vi "PostCopyScripting.vi"(10 "MetaDataObj":refnum<class "MetaDataObj.lvclass">, 11 "User Project":refnum<vi>) -> ()   [LabVIEW 2013, in "FixedChannelTBModuleDecideFeatures.lvclass"]
uses:
  FixedChannelTBModuleDecideFeatures.lvclass
  <resource>/dialog/NewProjectWizard/MetaDataObj/MetaDataObj.lvclass
  FixedChannelTBModuleDecideFeatures.lvclass/FixedChannelTBModuleDecideFeatures.ctl
  Read component name.vi
  Read Channel Specification.vi
  <resource>/dialog/NewProjectWizard/MetaDataObj/Accessors/Read Project Path.vi
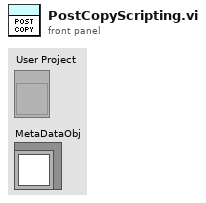
[diagram p1: front panel]
types:
  T1 = typedef "channel configuration.ctl" = cluster{"Name":string, "channel classification":T2, "data type":T3}
  T2 = typedef "TBM channel.lvclass/channel classification.ctl" = enum16{"input data", "output data", "processing parameter", "processing result"}
  T3 = typedef "tag bus.lvlib/tag descriptor.lvclass/Data Type.ctl" = enum16{"Double", "Single", "I64", "I32", "I16", "I8", "U64", "U32", "U16", "U8", "Boolean", "String", "Array of Double", "Array of Single", "Array of I64", "Array of I32", "Array of I16", "Array of I8", "Array of U64", "Array of U32", "Array of U16", "Array of U8", "Array of Boolean", "Array of String"}
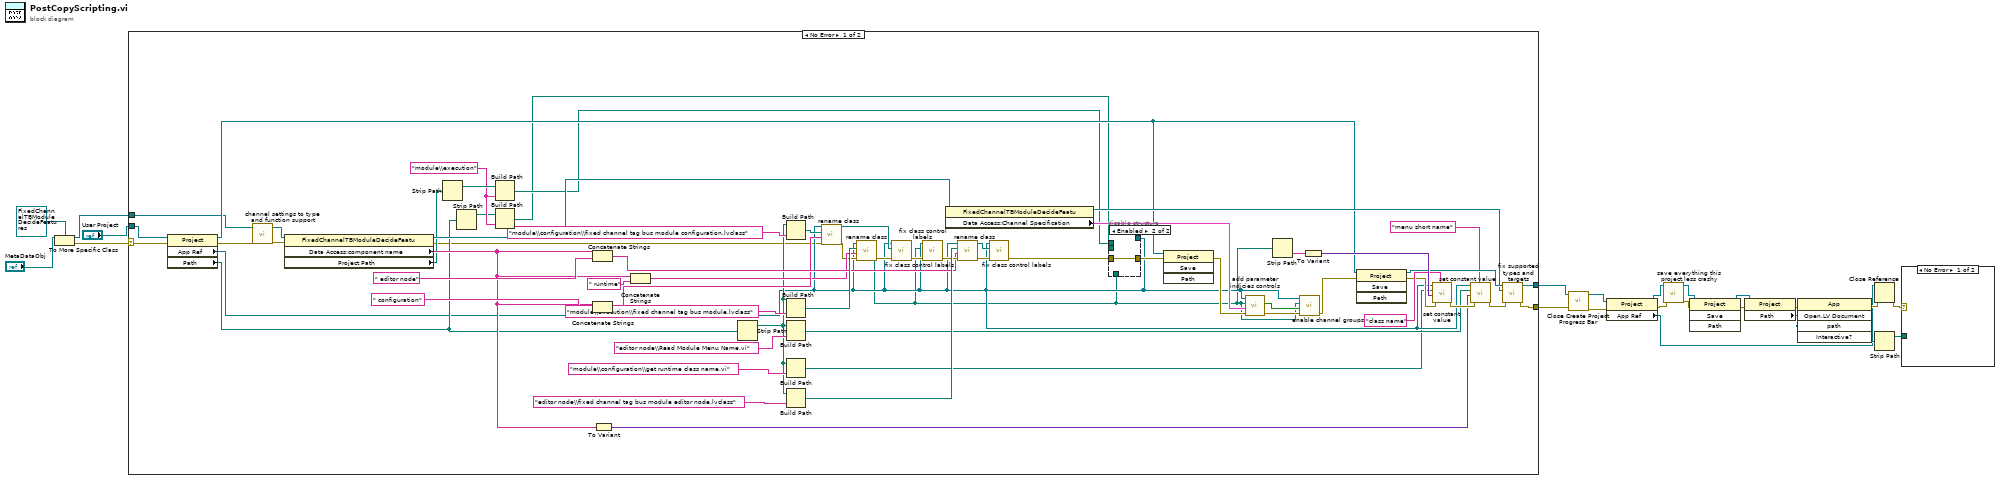
[diagram p0: block diagram]
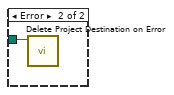
[diagram p2: hidden frame]
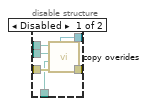
[diagram p3: hidden frame]
diagram:
  n1 = To More Specific Class(target class=refnum<class "FixedChannelTBModuleDecideFeatures.lvclass"> refnum ("DecideProjectFeatures.lvclass"), reference="MetaDataObj") -> (specific class reference=w12:refnum<class "FixedChannelTBModuleDecideFeatures.lvclass">, error out=w19:errorcluster)  [unwired: 1 in]
  n2 = case shown="No Error" w19 {
    selector: w19 -> [w24 w91]
    tunnel: [w63 w92] -> w1
    tunnel: "User Project" -> [w23 w92]
    tunnel: [w64 w91] -> w4
    tunnel: w12 -> [w26 _]
    frame No Error {
      w39 = "module\\execution"
      n3 = property class="Project"(reference=w23, error in=w24) -> (reference out=w42:refnum<vi>, error out=w25:errorcluster, "App Ref"=w31:refnum<vi>, "Path"=w37:path)
      n4 = call "channel settings to type and function support.vi"("error in"=w25, "FixedChannelTBModuleDecideFeatures in"=w26) -> ("error out"=w28:errorcluster, "FixedChannelTBModuleDecideFeatures out"=w27:refnum<class "FixedChannelTBModuleDecideFeatures.lvclass">)  [unwired: 8 in]
      n5 = property class="FixedChannelTBModuleDecideFeatu"(reference=w27, error in=w28) -> (reference out=w79:refnum<class "FixedChannelTBModuleDecideFeatures.lvclass">, error out=w29:errorcluster, "Data Access:component name"=w51:string, "Project Path"=w41:path)
      n6 = Strip Path(path=w41) -> (stripped path=w40:path)  [unwired: 1 out]
      n7 = Strip Path(path=w37) -> (stripped path=w36:path)  [unwired: 1 out]
      n8 = Build Path(base path=w40, name or relative path=w39) -> (appended path=w38:path)
      n9 = Build Path(base path=w36, name or relative path=w39) -> (appended path=w34:path)
      n10 = Concatenate Strings(w51, " editor node" ("string")) -> (w65:string)
      n11 = Concatenate Strings(w51, " configuration" ("string")) -> (w61:string)
      n12 = To Variant(anything=w51) -> (Variant=w57:variant)
      n13 = Concatenate Strings(w51, " runtime" ("string")) -> (w53:string)
      n14 = Strip Path(path=w37) -> (stripped path=w52:path)  [unwired: 1 out]
      n15 = Build Path(base path=w52, name or relative path="module\\configuration\\fixed channel tag bus module configuration.lvclass") -> (appended path=w49:path)
      n16 = Build Path(base path=w52, name or relative path="module\\execution\\fixed channel tag bus module.lvclass") -> (appended path=w81:path)
      n17 = Build Path(base path=w52, name or relative path="editor node\\Read Module Menu Name.vi") -> (appended path=w55:path)
      n18 = Build Path(base path=w52, name or relative path="module\\configuration\\get runtime class name.vi") -> (appended path=w22:path)
      n19 = Build Path(base path=w52, name or relative path="editor node\\fixed channel tag bus module editor node.lvclass") -> (appended path=w70:path)
      n20 = call "rename class.vi"("error in"=w29, "new name"=w61, "class path"=w49, "Application in"=w31) -> ("error out"=w50:errorcluster, "New Library Path"=w48:path)  [unwired: 6 in]
      n21 = call "rename class.vi"("error in"=w50, "new name"=w53, "class path"=w81, "Application in"=w31) -> ("error out"=w73:errorcluster, "New Library Path"=w30:path)  [unwired: 6 in]
      n22 = call "fix class control labels.vi"("error in"=w73, "class to load"=w48, "Application in"=w31) -> ("error out"=w72:errorcluster)  [unwired: 8 in]
      n23 = call "fix class control labels.vi"("error in"=w72, "class to load"=w30, "Application in"=w31) -> ("error out"=w67:errorcluster)  [unwired: 8 in]
      n24 = property class="FixedChannelTBModuleDecideFeatu"(reference=w79) -> (reference out=w47:refnum<class "FixedChannelTBModuleDecideFeatures.lvclass">, "Data Access:Channel Specification"=w46:T1[])  [unwired: 1 in, 1 out]
      n25 = call "rename class.vi"("error in"=w67, "new name"=w65, "class path"=w70, "Application in"=w31) -> ("error out"=w68:errorcluster, "New Library Path"=w69:path)  [unwired: 6 in]
      n26 = call "fix class control labels.vi"("error in"=w68, "class to load"=w69, "Application in"=w31) -> ("error out"=w32:errorcluster)  [unwired: 8 in]
      n27 = disable-structure shown="Enabled" {
        disable-tunnel: w38 -> [w89 _]
        disable-tunnel: w34 -> [w88 _]
        disable-tunnel: [w87 w90] -> w33
        disable-tunnel: w32 -> [w86 w90]
        disable-tunnel: w31 -> [w85 _]
        disable-tunnel: w30 -> [w84 _]
        frame Disabled {
          n28 = call "copy overides.vi"("application reference (local)"=w85, "error in"=w86, "New class path"=w84, "New path"=w88, "Old Path"=w89) -> ("error out"=w87:errorcluster)  [unwired: 6 in]
        }
        frame Enabled {
        }
      }
      n29 = invoke class="Project" method="Save"(reference=w42, error in=w33) -> (error out=w45:errorcluster)  [unwired: 2 in, 3 out]
      n30 = call "add parameter indicies controls.vi"("error in"=w45, "Channels to create"=w46, "class path"=w30, "Application in"=w31) -> ("error out"=w44:errorcluster, "Disable Channel Group?"=w43:bool[])  [unwired: 6 in]
      n31 = Strip Path(path=w30) -> (name=w60:string)  [unwired: 1 out]
      n32 = call "enable channel groups.vi"("error in"=w44, "Disable channel group?"=w43, "class path"=w30, "Application in"=w31) -> ("error out"=w35:errorcluster)  [unwired: 7 in]
      n33 = To Variant(anything=w60) -> (Variant=w78:variant)
      n34 = invoke class="Project" method="Save"(reference=w42, error in=w35) -> (reference out=w74:refnum<vi>, error out=w75:errorcluster)  [unwired: 2 in, 2 out]
      n35 = call "set constant value.vi"("control name"="class name", "error in"=w75, "data to set"=w78, "vi path"=w22, "Application in"=w31) -> ("error out"=w62:errorcluster)  [unwired: 6 in]
      n36 = call "set constant value.vi"("control name"="menu short name", "error in"=w62, "data to set"=w57, "vi path"=w55, "Application in"=w31) -> ("error out"=w59:errorcluster)  [unwired: 6 in]
      n37 = call "fix supported types and targets.vi"("error in"=w59, "DecideProjectFeatures in"=w47, "User Project in"=w74) -> ("error out"=w64:errorcluster, "User Project out"=w63:refnum<vi>)  [unwired: 7 in]
    }
    frame Error {
    }
  }
  n38 = call <resource>:"Close Create Project Progress Bar.vi"("error in (no error)"=w4, "Project"=w1) -> ("error out"=w3:errorcluster, "dup Project"=w2:refnum<vi>)  [unwired: 8 in]
  n39 = property class="Project"(reference=w2, error in=w3) -> (reference out=w9:refnum<vi>, error out=w10:errorcluster, "App Ref"=w8:refnum<vi>)
  n40 = call "save everything this project less crashy.vi"("error in"=w10, "Project in"=w9) -> ("error out"=w5:errorcluster, "Project out"=w11:refnum<vi>)  [unwired: 8 in]
  n41 = invoke class="Project" method="Save"(reference=w11, error in=w5) -> (reference out=w15:refnum<vi>, error out=w16:errorcluster)  [unwired: 2 in, 2 out]
  n42 = property class="Project"(reference=w15, error in=w16) -> (error out=w18:errorcluster, "Path"=w13:path)  [unwired: 1 out]
  n43 = invoke class="App" method="Open.LV Document"(error in=w18, "path"=w13) -> (error out=w17:errorcluster)  [unwired: 3 in, 4 out]
  n44 = Close Reference(reference=w8, error in (no error)=w17) -> (error out=w7:errorcluster)
  n45 = Strip Path(path=w13) -> (stripped path=w6:path)  [unwired: 1 out]
  n46 = case shown="No Error" w7 {
    tunnel: w6 -> [_ w93]
    frame No Error {
    }
    frame Error {
      n47 = call <resource>:"Delete Project Destination on Error.vi"("Project Destination Root"=w93) -> ()  [unwired: 11 in]
    }
  }
